vi "processCommands.vi"(8 "error in (no error)":errorcluster, 10 "commandKey":refnum<vi>, 11 "CommandProcessor in":refnum<class "CommandProcessor.lvclass">) -> (0 "error out":errorcluster, 3 "CommandProcessor out":refnum<class "CommandProcessor.lvclass">)   [LabVIEW 2011, in "Tools.lvlib" / "Interpreters.lvlib" / "CommandProcessor.lvclass"]
uses:
  CommandProcessor.lvclass
  CommandProcessor.lvclass/CommandProcessor.ctl
  SettingsEventManager/SettingsEventsManager.lvclass
  CommandEvents/CommandEvents.lvclass
  SettingsViewer/settingsViewer.lvclass
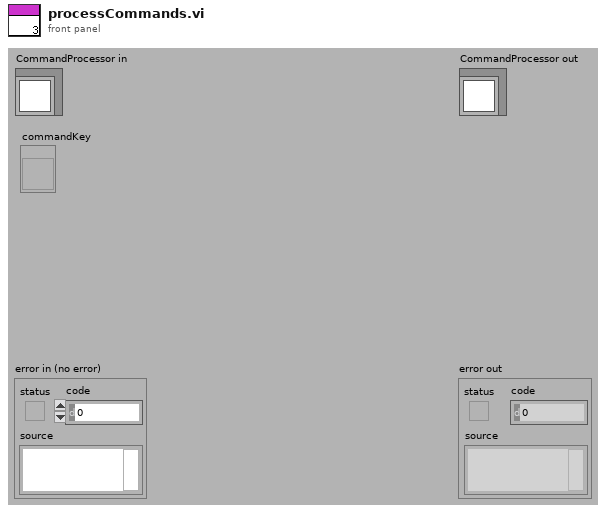
[diagram p1: front panel]
types:
  T1 = enum16{"Number", "String", "NumberArray", "StringArray"}
  T2 = enum16{"Number", "String", "NumberArray", "StringArray", "xmlNode"}
  T3 = cluster{"newCommand":refnum<user-event>, "textUpdate":refnum<user-event>}
  T4 = cluster{"settingsFrontEndEvents":cluster{"loadSettingsFromPath":refnum<user-event>, "lookUpElementEvent":refnum<user-event>, "saveSettings":refnum<user-event>, "loadSettings":refnum<user-event>, "close":refnum<user-event>, "replaceElement":refnum<user-event>, "findParentNodes":refnum<user-event>, "createNode":refnum<user-event>}, "settingBackEndEvents":cluster{"defaultSettingsPathRequest":refnum<user-event>, "searchResultEvent":refnum<user-event>, "settingsSaved":refnum<user-event>, "settingsLoaded":refnum<user-event>, "foundParentNode":refnum<user-event>}}
  T5 = enum16{"load;", "lookup;", "replace;", "save;", "close;", "use;", "nodePath;", "valuePath;", "?;", "info;", "insertNode;"}
  T6 = cluster{"loadSettingsFromPath":refnum<user-event>, "lookUpElementEvent":refnum<user-event>, "saveSettings":refnum<user-event>, "loadSettings":refnum<user-event>, "close":refnum<user-event>, "replaceElement":refnum<user-event>, "findParentNodes":refnum<user-event>, "createNode":refnum<user-event>}
  T7 = cluster{"element":string, string, "typeEnum":enum16{"Number", "String", "NumberArray", "StringArray"}}
  T8 = cluster{"element":string, "String":string, "typeEnum":enum16{"Number", "String", "NumberArray", "StringArray", "xmlNode"}}
  T9 = cluster{"element":string, string, "typeEnum":enum16{"Number", "String", "NumberArray", "StringArray", "xmlNode"}}
  T10 = cluster{"element":string, "String":string, "String":string}
  T11 = cluster{"element":string, "type":enum16{"element", "attribute", "value"}, "String":string}
  T12 = cluster{"element":string, "type":enum16{"element", "attribute", "value"}, string}
  T13 = cluster{string, string, "typeEnum":enum16{"Number", "String", "NumberArray", "StringArray", "xmlNode"}}
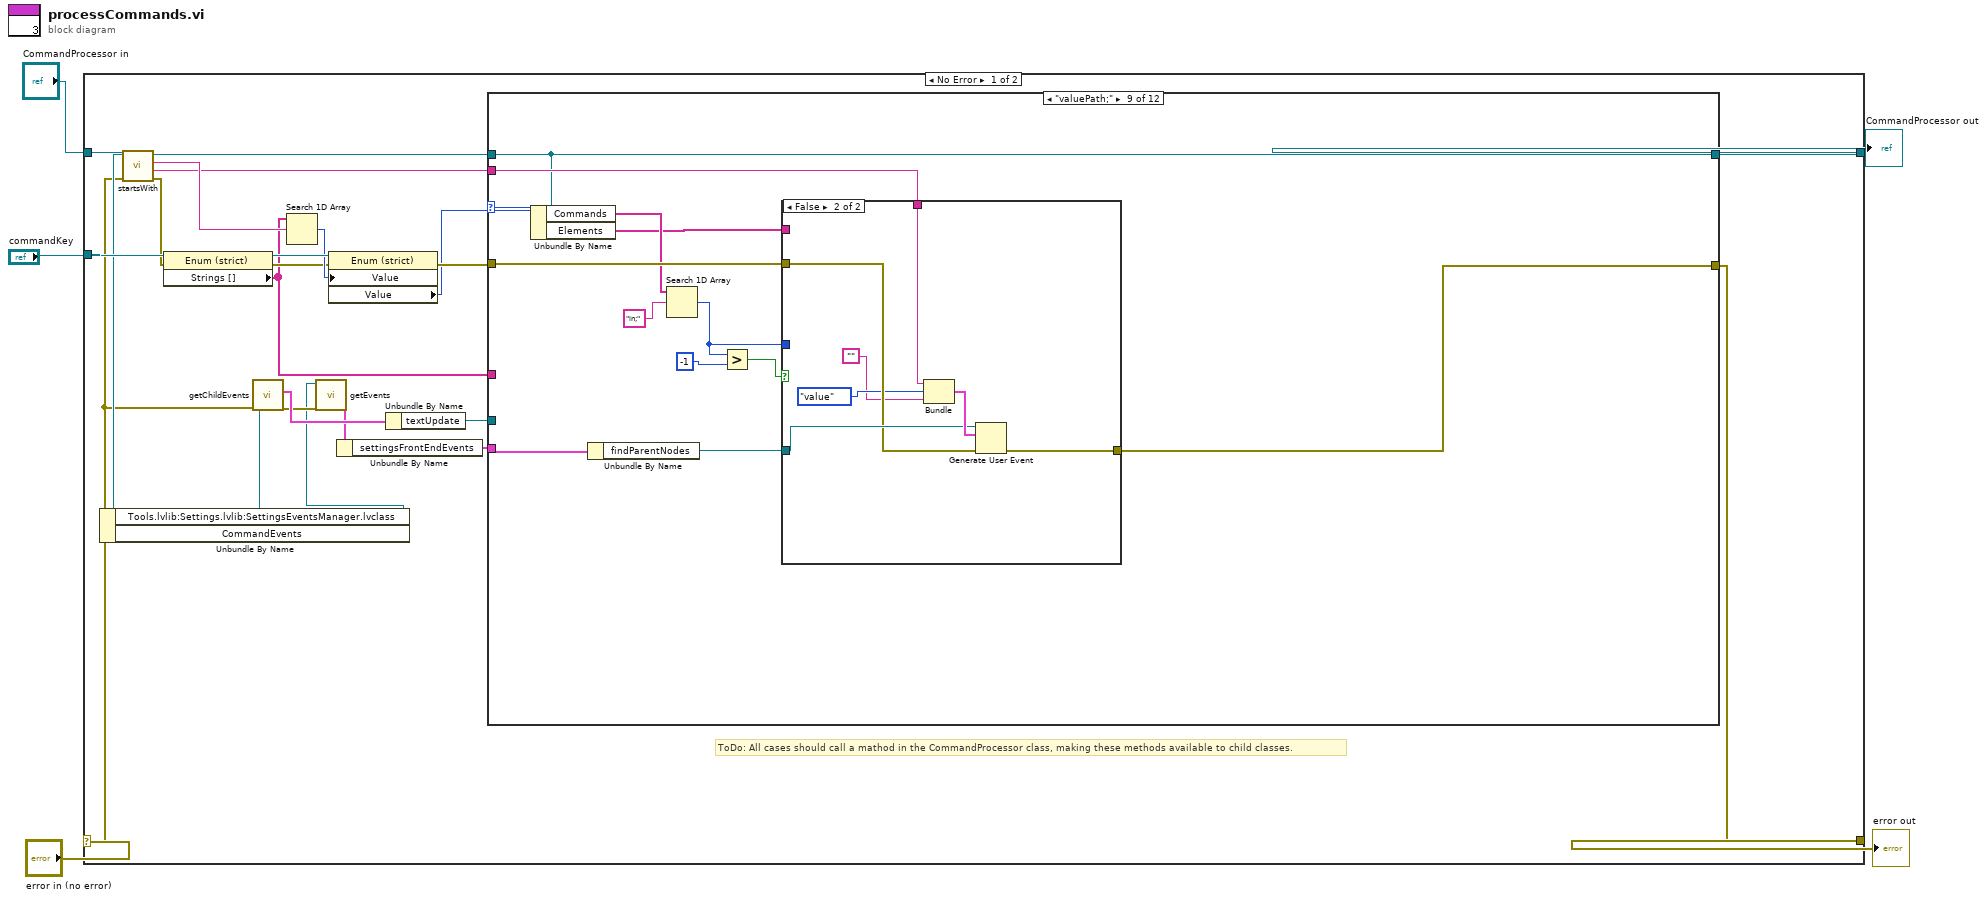
[diagram p0: block diagram]
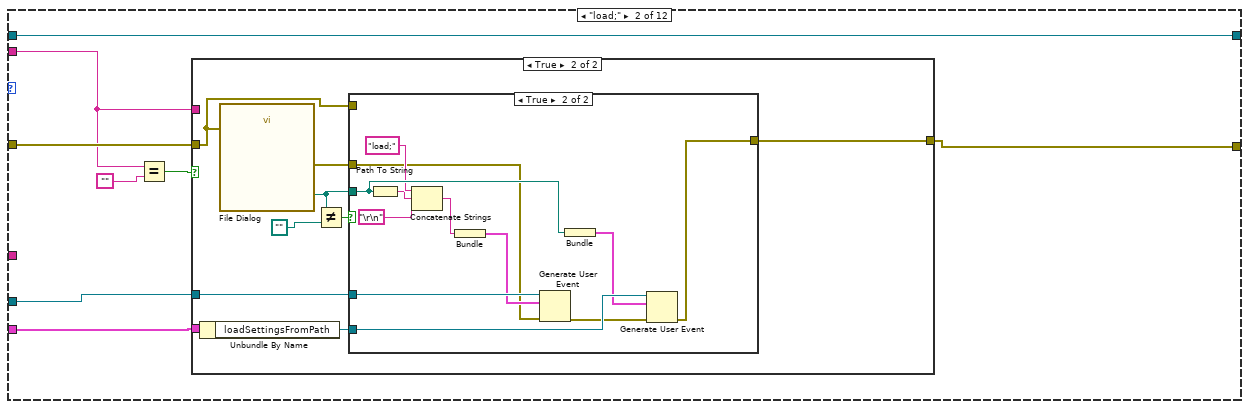
[diagram p3: hidden frame]
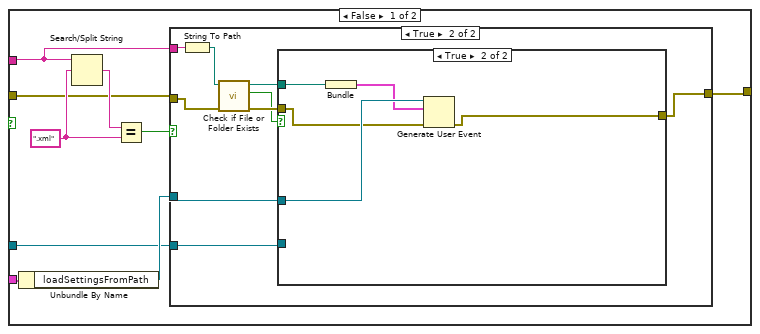
[diagram p4: hidden frame]
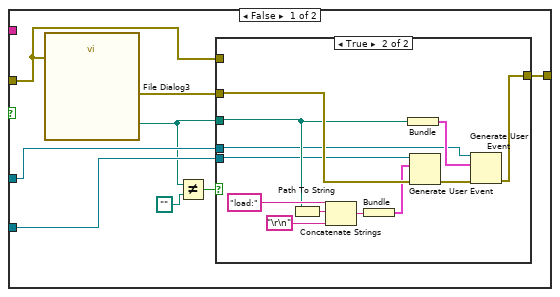
[diagram p5: hidden frame]
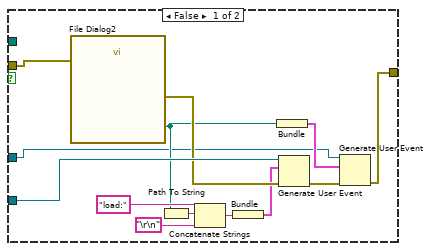
[diagram p7: hidden frame]
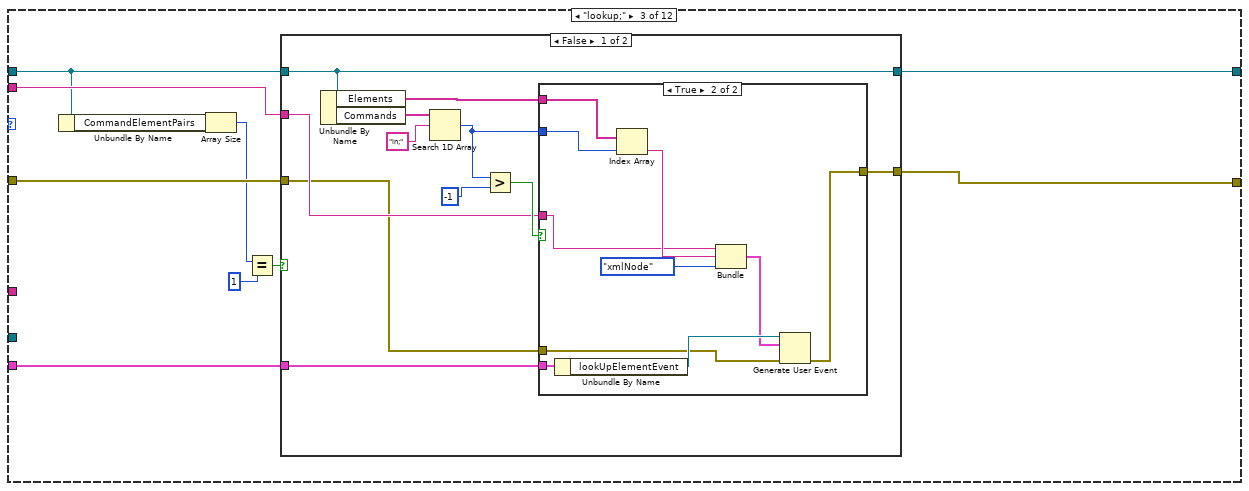
[diagram p9: hidden frame]
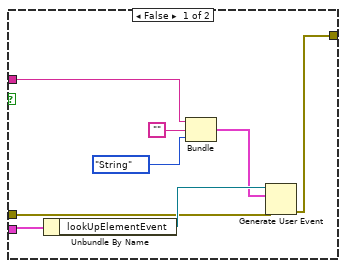
[diagram p10: hidden frame]
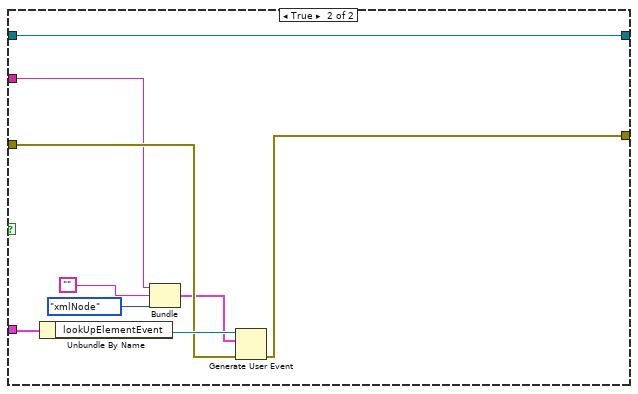
[diagram p11: hidden frame]
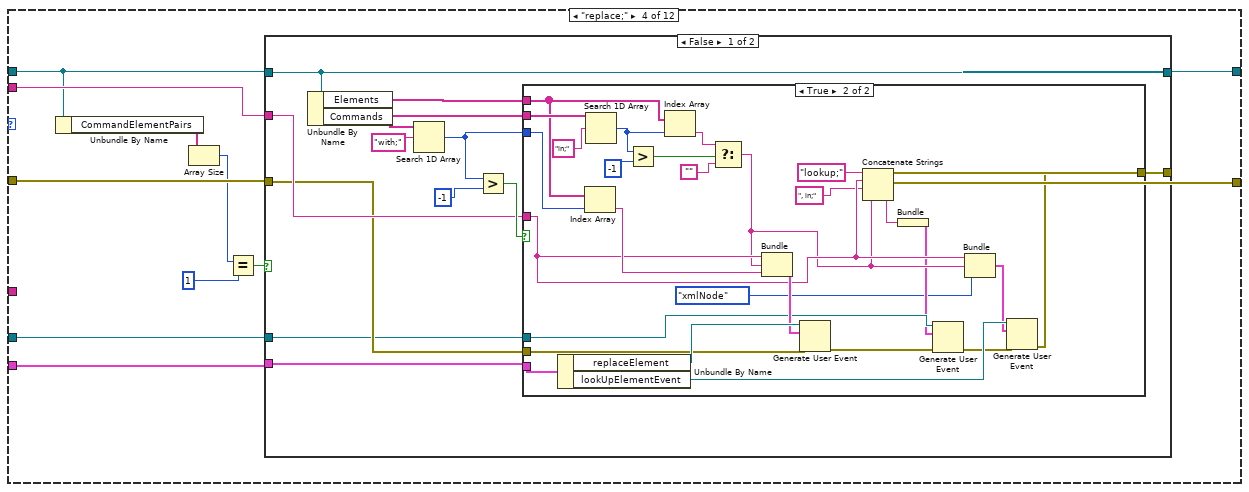
[diagram p12: hidden frame]
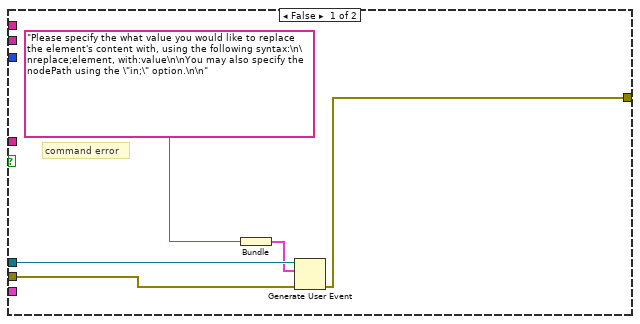
[diagram p13: hidden frame]
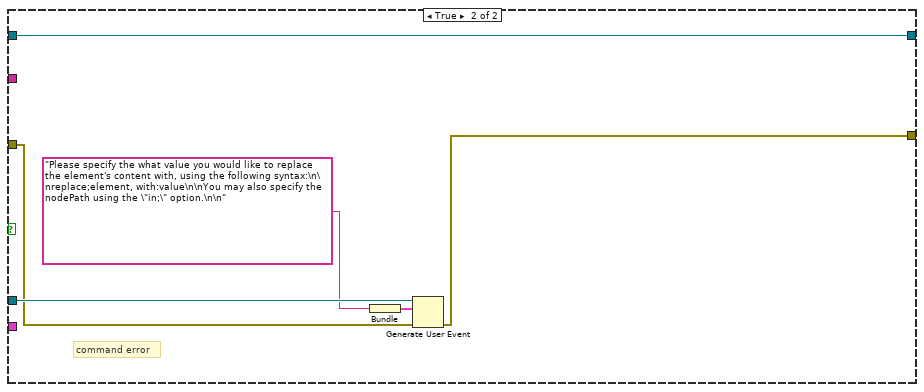
[diagram p14: hidden frame]
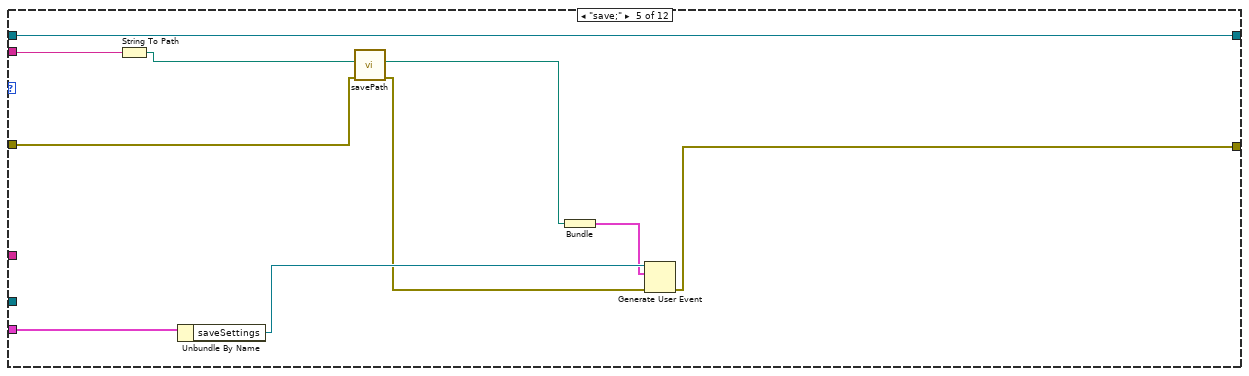
[diagram p15: hidden frame]
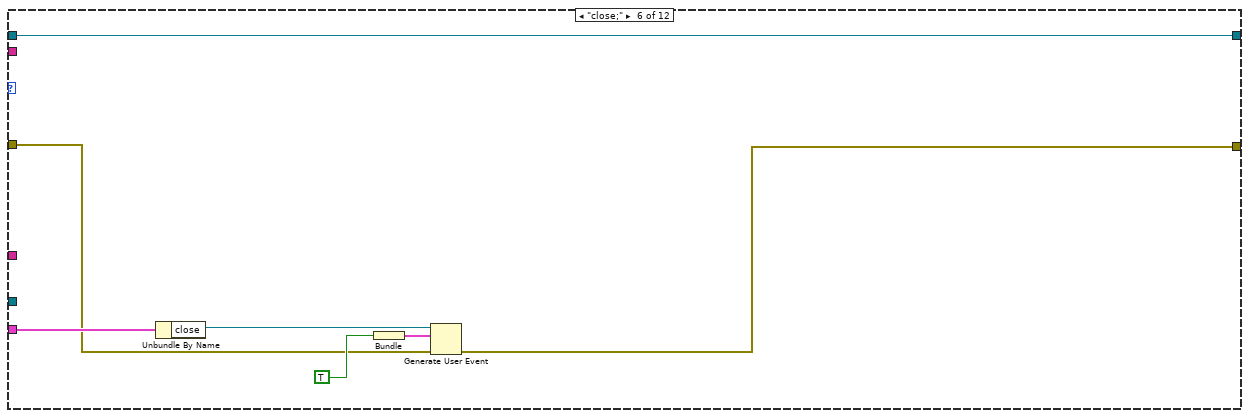
[diagram p16: hidden frame]
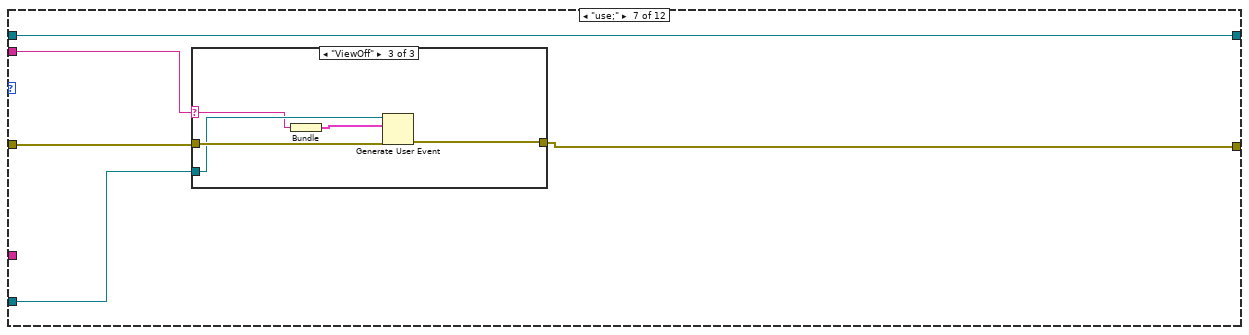
[diagram p17: hidden frame]
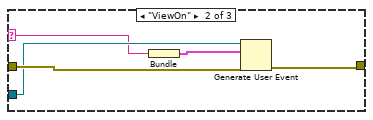
[diagram p19: hidden frame]
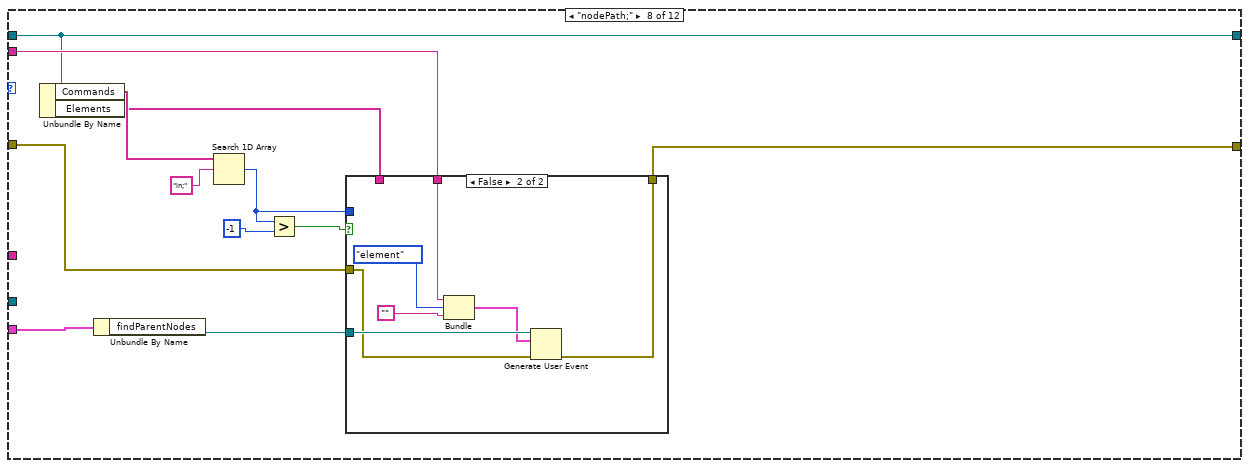
[diagram p20: hidden frame]
diagram:
  n1 = case shown="No Error" "error in (no error)" {
    selector: "error in (no error)" -> [w16 w404]
    tunnel: [w13 w404] -> w4
    tunnel: [w19 w403] -> w2
    tunnel: "CommandProcessor in" -> [w26 w403]
    tunnel: "commandKey" -> [w27 _]
    frame No Error {
      # "ToDo: All cases should call a mathod in the CommandProcessor class, making these methods available to child classes."
      n2 = call-dynamic "startsWith.vi"("error in (no error)"=w16, "CommandProcessor in"=w26) -> ("error out"=w25:errorcluster, "element"=w20:string, "command"=w24:string, "CommandProcessor out"=w18:refnum<class "CommandProcessor.lvclass">)  [unwired: 6 in]
      n3 = Unbundle By Name(w18) -> ("Tools.lvlib:Settings.lvlib:SettingsEventsManager.lvclass"=w7:refnum<class "SettingsEventsManager.lvclass">, "CommandEvents"=w17:refnum<class "CommandEvents.lvclass">)
      n4 = property class="Enum (strict)"(reference=w27, error in=w25) -> (reference out=w23:refnum<vi>, error out=w21:errorcluster, "Strings []"=w12:string[])
      n5 = call-dynamic "getChildEvents.vi"("error in (no error)"=w16, "CommandEvents in"=w17) -> ("error out"=w8:errorcluster, "Events"=w9:T3)  [unwired: 7 in, 1 out]
      n6 = Search 1D Array(1D array=w12, element=w24) -> (index of element=w22:i32)  [unwired: 1 in]
      n7 = call-dynamic "getEvents.vi"("error in (no error)"=w8, "SettingsEventsManager in"=w7) -> ("settingsEvents"=w6:T4)  [unwired: 7 in, 2 out]
      n8 = property class="Enum (strict)"(reference=w23, error in=w21, "Value"=w22) -> (error out=w11:errorcluster, "Value"=w10:T5)  [unwired: 1 out]
      n9 = Unbundle By Name(w6) -> ("settingsFrontEndEvents"=w14:T6)
      n10 = Unbundle By Name(w9) -> ("textUpdate"=w15:refnum<user-event>)
      n11 = case shown="\"valuePath;\"" w10 {
        tunnel: w18 -> [w29 w37 w117 w172 w235 w242 w247 w263 w293 w326 w332 w347]
        tunnel: w20 -> [_ w30 w120 w173 w234 _ w246 w267 w298 _ _ w346]
        tunnel: w11 -> [w28 w34 w126 w175 w232 w236 w244 w268 w295 w317 w334 w345]
        tunnel: [w29 w37 w118 w166 w235 w242 w247 w263 w293 w326 w332 w341] -> w19
        tunnel: w15 -> [_ w33 _ w165 _ _ w245 _ _ w320 _ w344]
        tunnel: w14 -> [_ w32 w121 w168 w231 w241 _ w270 w297 _ w340 w343]
        tunnel: [w28 w31 w119 w167 w226 w237 w243 w266 w294 w316 w333 w342] -> w13
        tunnel: w12 -> [_ _ _ _ _ _ _ _ _ w325 _ _]
        frame Default {
        }
        frame "load;" {
          n12 = Equal?(x=w30, y="") -> (x = y?=w36:bool)
          n13 = case shown="True" w36 {
            tunnel: w34 -> [w42 w96]
            tunnel: w33 -> [w38 w103]
            tunnel: w32 -> [w40 w101]
            tunnel: [w41 w99] -> w31
            tunnel: w30 -> [w43 _]
            frame False {
              w45 = ".xml"
              n14 = Unbundle By Name(w40) -> ("loadSettingsFromPath"=w39:refnum<user-event>)
              n15 = Search/Split String(string=w43, search string/char (-)=w45) -> (match + rest of string=w46:string)  [unwired: 1 in, 2 out]
              n16 = Equal?(x=w46, y=w45) -> (x = y?=w44:bool)
              n17 = case shown="True" w44 {
                tunnel: w43 -> [_ w76]
                tunnel: w42 -> [w48 w74]
                tunnel: [w51 w69] -> w41
                tunnel: w39 -> [w53 w71]
                tunnel: w38 -> [w52 w68]
                frame False {
                  n18 = call "File Dialog3"("error in"=w48) -> ("selected path"=w49:path, "error out"=w54:errorcluster)  [unwired: 11 in, 2 out]
                  n19 = Not Equal?(x=w49, y=path "") -> (x != y?=w50:bool)
                  n20 = case shown="True" w50 {
                    tunnel: w54 -> [_ w66]
                    tunnel: w49 -> [_ w62]
                    tunnel: w53 -> [_ w58]
                    tunnel: w52 -> [_ w57]
                    tunnel: [w55 w56] -> w51
                    tunnel: w48 -> [w55 _]
                    frame False {
                    }
                    frame True {
                      n21 = Path To String(path=w62) -> (string=w63:string)
                      n22 = Concatenate Strings("load:", w63, "\r\n") -> (w61:string)
                      n23 = Bundle(w61) -> (w60:cluster{string})  [unwired: 1 in]
                      n24 = Bundle("selected path"=w62) -> (w67:cluster{"selected path":path})  [unwired: 1 in]
                      n25 = Generate User Event(user event=w57, event data cluster=w60, error in=w66) -> (error out=w59:errorcluster)  [unwired: 1 out]
                      n26 = Generate User Event(user event=w58, event data cluster=w67, error in=w59) -> (error out=w56:errorcluster)  [unwired: 1 out]
                    }
                  }
                }
                frame True {
                  n27 = String To Path(string=w76) -> (path=w75:path)
                  n28 = call <vilib>:"Check if File or Folder Exists.vi"("error in (no error)"=w74, "path"=w75) -> ("error out"=w73:errorcluster, "file or folder exists?"=w72:bool, "dup path"=w70:path)  [unwired: 7 in]
                  n29 = case shown="True" w72 {
                    tunnel: w73 -> [w89 w91]
                    tunnel: w71 -> [w78 w94]
                    tunnel: w70 -> [_ w93]
                    tunnel: [w77 w90] -> w69
                    tunnel: w68 -> [w87 _]
                    frame False {
                      n30 = call "File Dialog2"("error in"=w89) -> ("selected path"=w82:path, "error out"=w86:errorcluster)  [unwired: 11 in, 2 out]
                      n31 = Path To String(path=w82) -> (string=w83:string)
                      n32 = Concatenate Strings("load:", w83, "\r\n") -> (w81:string)
                      n33 = Bundle(w81) -> (w80:cluster{string})  [unwired: 1 in]
                      n34 = Bundle("selected path"=w82) -> (w88:cluster{"selected path":path})  [unwired: 1 in]
                      n35 = Generate User Event(user event=w87, event data cluster=w80, error in=w86) -> (error out=w79:errorcluster)  [unwired: 1 out]
                      n36 = Generate User Event(user event=w78, event data cluster=w88, error in=w79) -> (error out=w77:errorcluster)  [unwired: 1 out]
                    }
                    frame True {
                      n37 = Bundle("dup path"=w93) -> (w92:cluster{"dup path":path})  [unwired: 1 in]
                      n38 = Generate User Event(user event=w94, event data cluster=w92, error in=w91) -> (error out=w90:errorcluster)  [unwired: 1 out]
                    }
                  }
                }
              }
            }
            frame True {
              n39 = Unbundle By Name(w101) -> ("loadSettingsFromPath"=w100:refnum<user-event>)
              n40 = call "File Dialog"("error in"=w96) -> ("selected path"=w97:path, "error out"=w102:errorcluster)  [unwired: 11 in, 2 out]
              n41 = Not Equal?(x=w97, y=path "") -> (x != y?=w98:bool)
              n42 = case shown="True" w98 {
                tunnel: w103 -> [_ w115]
                tunnel: w102 -> [_ w105]
                tunnel: w100 -> [_ w112]
                tunnel: w97 -> [_ w110]
                tunnel: [w104 w108] -> w99
                tunnel: w96 -> [w104 _]
                frame False {
                }
                frame True {
                  n43 = Path To String(path=w110) -> (string=w106:string)
                  n44 = Concatenate Strings("load;", w106, "\r\n") -> (w114:string)
                  n45 = Bundle(w114) -> (w113:cluster{string})  [unwired: 1 in]
                  n46 = Generate User Event(user event=w115, event data cluster=w113, error in=w105) -> (error out=w111:errorcluster)  [unwired: 1 out]
                  n47 = Bundle("selected path"=w110) -> (w109:cluster{"selected path":path})  [unwired: 1 in]
                  n48 = Generate User Event(user event=w112, event data cluster=w109, error in=w111) -> (error out=w108:errorcluster)  [unwired: 1 out]
                }
              }
            }
          }
        }
        frame "lookup;" {
          n49 = Unbundle By Name(w117) -> ("CommandElementPairs"=w122:string[])
          n50 = Array Size(array=w122) -> (size(s)=w124:i32)
          n51 = Equal?(x=w124, y=1) -> (x = y?=w125:bool)
          n52 = case shown="False" w125 {
            tunnel: w126 -> [w128 w162]
            tunnel: w121 -> [w130 w164]
            tunnel: w120 -> [w129 w161]
            tunnel: [w127 w157] -> w119
            tunnel: w117 -> [w137 w156]
            tunnel: [w137 w156] -> w118
            frame False {
              n53 = Unbundle By Name(w137) -> ("Elements"=w131:string[], "Commands"=w136:string[])
              n54 = Search 1D Array(1D array=w136, element="in;") -> (index of element=w132:i32)  [unwired: 1 in]
              n55 = Greater?(x=w132, y=-1) -> (0:w133:bool)
              n56 = case shown="True" w133 {
                tunnel: w132 -> [_ w154]
                tunnel: w131 -> [_ w155]
                tunnel: w130 -> [w145 w153]
                tunnel: w129 -> [w142 w149]
                tunnel: w128 -> [w143 w147]
                tunnel: [w138 w146] -> w127
                frame False {
                  n57 = Unbundle By Name(w145) -> ("lookUpElementEvent"=w144:refnum<user-event>)
                  n58 = Bundle("element"=w142, "", "typeEnum"=T1."String") -> (w139:T7)  [unwired: 1 in]
                  n59 = Generate User Event(user event=w144, event data cluster=w139, error in=w143) -> (error out=w138:errorcluster)  [unwired: 1 out]
                }
                frame True {
                  n60 = Unbundle By Name(w153) -> ("lookUpElementEvent"=w152:refnum<user-event>)
                  n61 = Index Array(array=w155, index=w154) -> (element=w150:string)
                  n62 = Bundle("element"=w149, "String"=w150, "typeEnum"=T2."xmlNode") -> (w148:T8)  [unwired: 1 in]
                  n63 = Generate User Event(user event=w152, event data cluster=w148, error in=w147) -> (error out=w146:errorcluster)  [unwired: 1 out]
                }
              }
            }
            frame True {
              n64 = Unbundle By Name(w164) -> ("lookUpElementEvent"=w163:refnum<user-event>)
              n65 = Bundle("element"=w161, "", "typeEnum"=T2."xmlNode") -> (w158:T9)  [unwired: 1 in]
              n66 = Generate User Event(user event=w163, event data cluster=w158, error in=w162) -> (error out=w157:errorcluster)  [unwired: 1 out]
            }
          }
        }
        frame "replace;" {
          n67 = Unbundle By Name(w172) -> ("CommandElementPairs"=w174:string[])
          n68 = Array Size(array=w174) -> (size(s)=w170:i32)
          n69 = Equal?(x=w170, y=1) -> (x = y?=w169:bool)
          n70 = case shown="False" w169 {
            tunnel: w175 -> [w180 w221]
            tunnel: w173 -> [w181 _]
            tunnel: [w179 w220] -> w167
            tunnel: w172 -> [w187 w225]
            tunnel: [w187 w225] -> w166
            tunnel: w168 -> [w178 _]
            tunnel: w165 -> [w177 w224]
            frame False {
              n71 = Unbundle By Name(w187) -> ("Elements"=w182:string[], "Commands"=w176:string[])
              n72 = Search 1D Array(1D array=w176, element="with;") -> (index of element=w183:i32)  [unwired: 1 in]
              n73 = Greater?(x=w183, y=-1) -> (0:w184:bool)
              n74 = case shown="True" w184 {
                tunnel: w183 -> [_ w209]
                tunnel: w182 -> [_ w206]
                tunnel: w178 -> [_ w219]
                tunnel: w181 -> [_ w201]
                tunnel: w180 -> [w189 w217]
                tunnel: [w188 w203] -> w179
                tunnel: w177 -> [w192 w196]
                tunnel: w176 -> [_ w208]
                frame False {
                  # "command error"
                  n75 = Bundle("Please specify the what value you would like to replace the element's content with, using the following syntax:\n\nreplace;element, with:value\n\nYou may also specify the nodePath using the \"in;\" option.\n\n") -> (w190:cluster{string})  [unwired: 1 in]
                  n76 = Generate User Event(user event=w192, event data cluster=w190, error in=w189) -> (error out=w188:errorcluster)  [unwired: 1 out]
                }
                frame True {
                  n77 = Unbundle By Name(w219) -> ("replaceElement"=w218:refnum<user-event>, "lookUpElementEvent"=w205:refnum<user-event>)
                  n78 = Index Array(array=w206, index=w209) -> (element=w207:string)
                  n79 = Search 1D Array(1D array=w208, element="in;") -> (index of element=w211:i32)  [unwired: 1 in]
                  n80 = Greater?(x=w211, y=-1) -> (0:w213:bool)
                  n81 = Index Array(array=w206, index=w211) -> (element=w212:string)
                  n82 = Select(t=w212, s=w213, f="") -> (s? t:f=w199:string)
                  n83 = Bundle("element"=w201, "String"=w199, "String"=w207) -> (w216:T10)  [unwired: 1 in]
                  n84 = Generate User Event(user event=w218, event data cluster=w216, error in=w217) -> (error out=w198:errorcluster)  [unwired: 1 out]
                  n85 = Concatenate Strings("lookup;", w201, ", in;", w199) -> (w194:string)
                  n86 = Bundle(w194) -> (w195:cluster{string})  [unwired: 1 in]
                  n87 = Generate User Event(user event=w196, event data cluster=w195, error in=w198) -> (error out=w197:errorcluster)  [unwired: 1 out]
                  n88 = Bundle("element"=w201, "String"=w199, "typeEnum"=T2."xmlNode") -> (w204:T8)  [unwired: 1 in]
                  n89 = Generate User Event(user event=w205, event data cluster=w204, error in=w197) -> (error out=w203:errorcluster)  [unwired: 1 out]
                }
              }
            }
            frame True {
              # "command error"
              n90 = Bundle("Please specify the what value you would like to replace the element's content with, using the following syntax:\n\nreplace;element, with:value\n\nYou may also specify the nodePath using the \"in;\" option.\n\n") -> (w222:cluster{string})  [unwired: 1 in]
              n91 = Generate User Event(user event=w224, event data cluster=w222, error in=w221) -> (error out=w220:errorcluster)  [unwired: 1 out]
            }
          }
        }
        frame "save;" {
          n92 = String To Path(string=w234) -> (path=w233:path)
          n93 = Unbundle By Name(w231) -> ("saveSettings"=w230:refnum<user-event>)
          n94 = call "savePath.vi"("error in (no error)"=w232, "Path  in"=w233) -> ("error out"=w227:errorcluster, "Path out"=w229:path)  [unwired: 7 in, 1 out]
          n95 = Bundle("Path out"=w229) -> (w228:cluster{"Path out":path})  [unwired: 1 in]
          n96 = Generate User Event(user event=w230, event data cluster=w228, error in=w227) -> (error out=w226:errorcluster)  [unwired: 1 out]
        }
        frame "close;" {
          n97 = Unbundle By Name(w241) -> ("close"=w240:refnum<user-event>)
          n98 = Bundle(TRUE) -> (w238:cluster{bool})  [unwired: 1 in]
          n99 = Generate User Event(user event=w240, event data cluster=w238, error in=w236) -> (error out=w237:errorcluster)  [unwired: 1 out]
        }
        frame "use;" {
          n100 = case shown="\"ViewOff\"" w246 {
            selector: w246 -> [_ w250 w255]
            tunnel: w245 -> [_ w251 w257]
            tunnel: w244 -> [w248 w252 w258]
            tunnel: [w248 w249 w256] -> w243
            frame Default {
            }
            frame "ViewOn" {
              n101 = Bundle(w250) -> (w253:cluster{string})  [unwired: 1 in]
              n102 = Generate User Event(user event=w251, event data cluster=w253, error in=w252) -> (error out=w249:errorcluster)  [unwired: 1 out]
            }
            frame "ViewOff" {
              n103 = Bundle(w255) -> (w254:cluster{string})  [unwired: 1 in]
              n104 = Generate User Event(user event=w257, event data cluster=w254, error in=w258) -> (error out=w256:errorcluster)  [unwired: 1 out]
            }
          }
        }
        frame "nodePath;" {
          n105 = Unbundle By Name(w263) -> ("Commands"=w262:string[], "Elements"=w260:string[])
          n106 = Unbundle By Name(w270) -> ("findParentNodes"=w269:refnum<user-event>)
          n107 = Search 1D Array(1D array=w262, element="in;") -> (index of element=w259:i32)  [unwired: 1 in]
          n108 = Greater?(x=w259, y=-1) -> (0:w261:bool)
          n109 = case shown="False" w261 {
            tunnel: w269 -> [w279 w286]
            tunnel: w268 -> [w276 w283]
            tunnel: w267 -> [w275 w282]
            tunnel: [w274 w281] -> w266
            tunnel: w260 -> [w273 _]
            tunnel: w259 -> [w272 _]
            frame True {
              n110 = Index Array(array=w273, index=w272) -> (element=w271:string)
              n111 = Bundle("element"=w275, "type"=enum16{"element", "attribute", "value"}."element", "String"=w271) -> (w278:T11)  [unwired: 1 in]
              n112 = Generate User Event(user event=w279, event data cluster=w278, error in=w276) -> (error out=w274:errorcluster)  [unwired: 1 out]
            }
            frame False {
              n113 = Bundle("element"=w282, "type"=enum16{"element", "attribute", "value"}."element", "") -> (w285:T12)  [unwired: 1 in]
              n114 = Generate User Event(user event=w286, event data cluster=w285, error in=w283) -> (error out=w281:errorcluster)  [unwired: 1 out]
            }
          }
        }
        frame "valuePath;" {
          n115 = Unbundle By Name(w293) -> ("Commands"=w290:string[], "Elements"=w287:string[])
          n116 = Unbundle By Name(w297) -> ("findParentNodes"=w296:refnum<user-event>)
          n117 = Search 1D Array(1D array=w290, element="in;") -> (index of element=w288:i32)  [unwired: 1 in]
          n118 = Greater?(x=w288, y=-1) -> (0:w289:bool)
          n119 = case shown="False" w289 {
            tunnel: w298 -> [w306 w313]
            tunnel: w296 -> [w305 w312]
            tunnel: w295 -> [w304 w311]
            tunnel: [w302 w309] -> w294
            tunnel: w288 -> [w300 _]
            tunnel: w287 -> [w301 _]
            frame True {
              n120 = Index Array(array=w301, index=w300) -> (element=w299:string)
              n121 = Bundle("element"=w306, "type"=enum16{"element", "attribute", "value"}."value", "String"=w299) -> (w307:T11)  [unwired: 1 in]
              n122 = Generate User Event(user event=w305, event data cluster=w307, error in=w304) -> (error out=w302:errorcluster)  [unwired: 1 out]
            }
            frame False {
              n123 = Bundle("element"=w313, "type"=enum16{"element", "attribute", "value"}."value", "") -> (w314:T12)  [unwired: 1 in]
              n124 = Generate User Event(user event=w312, event data cluster=w314, error in=w311) -> (error out=w309:errorcluster)  [unwired: 1 out]
            }
          }
        }
        frame "?;" {
          n125 = for {
            tunnel: w325 -> [w329] mode=indexing
            shift-right: [w330] -> w322
            shift-left: "" -> [w331]
            n126 = call <vilib>:"Space Constant.vi"() -> ("String"=w327:string)
            n127 = Concatenate Strings(w327, w327, w327, w327, w327, w327, w327, w327, w327) -> (w328:string)
            n128 = Concatenate Strings(w331, w329, w328) -> (w330:string)
          }
          n129 = Concatenate Strings("The correct Command Syntax is of the form \"command;element\". For example, \"lookup;channel_number\".\n\nHere is a list of command you may use:\n", w322, "\r\n", "You may also use the following options:         in;         with;\nFor example:\n\nlookup;channel_number type=\"analog\", in;/device_settings/ao name=\"Ao8\"\n\nor,\n\nreplace;mappedTo type=\"magnetic_field\", in;/channel_config name=\"Ao8_00\"/mapping, with;Brf[G]\n\n") -> (w319:string)
          n130 = Bundle(w319) -> (w318:cluster{string})  [unwired: 1 in]
          n131 = Generate User Event(user event=w320, event data cluster=w318, error in=w317) -> (error out=w316:errorcluster)  [unwired: 1 out]
        }
        frame "info;" {
          # "This case should probably be in a child of the CommandProcessor class, but I haven't got round to making that yet."
          # "The database has a node called info, which contains information about the structure of the xml.\nThis shortcut command, requests this information."
          n132 = Unbundle By Name(w340) -> ("lookUpElementEvent"=w339:refnum<user-event>)
          n133 = Bundle("info", "/device_settings", "typeEnum"=T2."xmlNode") -> (w335:T13)  [unwired: 1 in]
          n134 = Generate User Event(user event=w339, event data cluster=w335, error in=w334) -> (error out=w333:errorcluster)  [unwired: 1 out]
        }
        frame "insertNode;" {
          n135 = Unbundle By Name(w347) -> ("CommandElementPairs"=w351:string[])
          n136 = Array Size(array=w351) -> (size(s)=w349:i32)
          n137 = Equal?(x=w349, y=1) -> (x = y?=w348:bool)
          n138 = case shown="False" w348 {
            tunnel: w345 -> [w356 w398]
            tunnel: w346 -> [w357 _]
            tunnel: [w355 w397] -> w342
            tunnel: w347 -> [w363 w402]
            tunnel: [w363 w402] -> w341
            tunnel: w343 -> [w354 _]
            tunnel: w344 -> [w353 w401]
            frame False {
              n139 = Unbundle By Name(w363) -> ("Elements"=w358:string[], "Commands"=w352:string[])
              n140 = Search 1D Array(1D array=w352, element="in;") -> (index of element=w359:i32)  [unwired: 1 in]
              n141 = Greater?(x=w359, y=-1) -> (0:w360:bool)
              n142 = case shown="True" w360 {
                tunnel: w359 -> [_ w392]
                tunnel: w358 -> [_ w391]
                tunnel: w354 -> [w367 w396]
                tunnel: w357 -> [w365 w393]
                tunnel: w356 -> [w369 w394]
                tunnel: [w368 w380] -> w355
                tunnel: w353 -> [_ w377]
                tunnel: w352 -> [_ _]
                frame False {
                  n143 = Unbundle By Name(w367) -> ("createNode"=w366:refnum<user-event>)
                  n144 = Bundle("element"=w365, "") -> (w370:cluster{"element":string, string})  [unwired: 1 in]
                  n145 = Generate User Event(user event=w366, event data cluster=w370, error in=w369) -> (error out=w368:errorcluster)  [unwired: 1 out]
                }
                frame True {
                  w386 = "/"
                  n146 = Unbundle By Name(w396) -> ("createNode"=w395:refnum<user-event>, "lookUpElementEvent"=w381:refnum<user-event>)
                  n147 = Index Array(array=w391, index=w392) -> (element=w389:string)
                  n148 = Reverse String(1:w389) -> (0:w388:string)
                  n149 = Bundle("element"=w393, "String"=w389) -> (w390:cluster{"element":string, "String":string})  [unwired: 1 in]
                  n150 = Search/Split String(string=w388, search string/char (-)=w386) -> (substring before match=w384:string, match + rest of string=w387:string)  [unwired: 1 in, 1 out]
                  n151 = Generate User Event(user event=w395, event data cluster=w390, error in=w394) -> (error out=w379:errorcluster)  [unwired: 1 out]
                  n152 = Search and Replace String(input string=w387, search string=w386) -> (result string=w385:string)  [unwired: 6 in, 3 out]
                  n153 = Reverse String(1:w384) -> (0:w375:string)
                  n154 = Reverse String(1:w385) -> (0:w373:string)
                  n155 = Bundle(w375, w373, "typeEnum"=T2."xmlNode") -> (w382:T13)  [unwired: 1 in]
                  n156 = Concatenate Strings("lookup;", w375, ", in;", w373) -> (w372:string)
                  n157 = Bundle(w372) -> (w371:cluster{string})  [unwired: 1 in]
                  n158 = Generate User Event(user event=w377, event data cluster=w371, error in=w379) -> (error out=w378:errorcluster)  [unwired: 1 out]
                  n159 = Generate User Event(user event=w381, event data cluster=w382, error in=w378) -> (error out=w380:errorcluster)  [unwired: 1 out]
                }
              }
            }
            frame True {
              # "command error"
              n160 = Bundle("Please specify the what value you would like to replace the element's content with, using the following syntax:\n\nreplace;element, with:value\n\nYou may also specify the nodePath using the \"in;\" option.\n\n") -> (w399:cluster{string})  [unwired: 1 in]
              n161 = Generate User Event(user event=w401, event data cluster=w399, error in=w398) -> (error out=w397:errorcluster)  [unwired: 1 out]
            }
          }
        }
      }
    }
    frame Error {
    }
  }
  "error out" <- w4
  "CommandProcessor out" <- w2
